vi "安装可执行文件并运行.vi"(8 "error in (no error)":errorcluster, 10 "目标路径（使用对话框）":path, 11 "源路径":path) -> (0 "error out":errorcluster)   [LabVIEW 2016, in "数据传输系统-03.lvlib" / "update.lvlib" / "http client.lvclass"]
uses:
  http client.lvclass
  update.lvlib
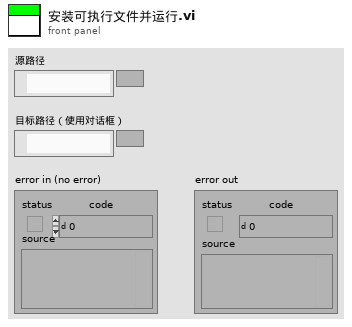
[diagram p1: front panel]
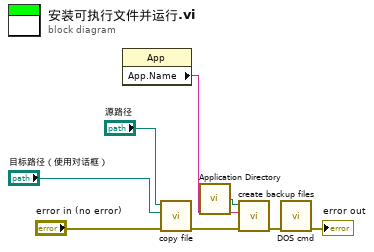
[diagram p0: block diagram]
diagram:
  n1 = property class="App"() -> ("App.Name"=w8:string)  [unwired: 2 in, 2 out]
  n2 = call "copy file.vi"("error in (no error)"="error in (no error)", "目标路径（使用对话框）"="目标路径（使用对话框）", "源路径"="源路径") -> ("error out"=w4:errorcluster)  [unwired: 8 in]
  n3 = call <vilib>:"Application Directory.vi"() -> ("Application Directory"=w1:path)
  n4 = call "create backup files.vi"("error in (no error)"=w4, "execute file name"=w8, "路径"=w1) -> ("error out"=w7:errorcluster)  [unwired: 8 in]
  n5 = call "DOS cmd.vi"("错误输入（无错误）"=w7) -> ("error out"=→"error out":errorcluster)  [unwired: 10 in]
